vi "average safe rate.vi"(8 "Back Right":dbl, 9 "Front Right":dbl, 10 "Back Left":dbl, 11 "Front Left":dbl) -> (0 "Right Average Rate":dbl, 3 "Left Average Rate":dbl)   [LabVIEW 2014]
panel:
  # "If the person reading this is Michael, haha too late, this was committed\n\nIf the person reading this isn't Michael, hello! From the past!"
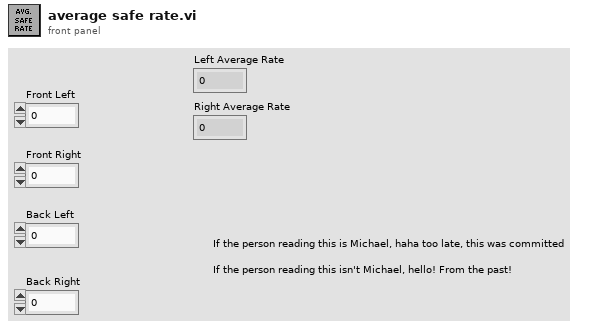
[diagram p1: front panel]
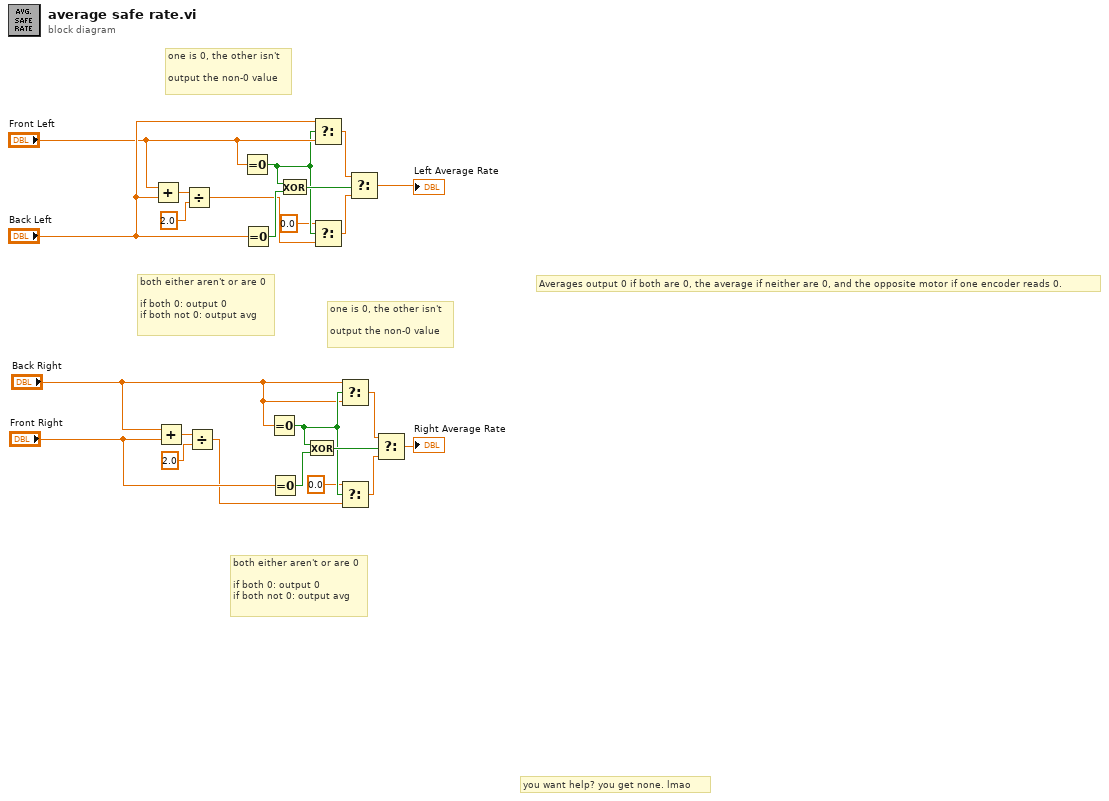
[diagram p0: block diagram]
diagram:
  # "one is 0, the other isn't\n\noutput the non-0 value"
  # "one is 0, the other isn't\n\noutput the non-0 value"
  # "both either aren't or are 0\n\nif both 0: output 0\nif both not 0: output avg"
  # "both either aren't or are 0\n\nif both 0: output 0\nif both not 0: output avg"
  # "Averages output 0 if both are 0, the average if neither are 0, and the opposite motor if one encoder reads 0."
  # "you want help? you get none. lmao"
  n1 = Add(x="Front Left", y="Back Left") -> (x+y=w24:dbl)
  n2 = Add(x="Back Right", y="Front Right") -> (x+y=w21:dbl)
  n3 = Divide(x=w24, y=2.0) -> (x/y=w12:dbl)
  n4 = Divide(x=w21, y=2.0) -> (x/y=w1:dbl)
  n5 = Equal To 0?(x="Front Left") -> (x = 0?=w14:bool)
  n6 = Equal To 0?(x="Back Left") -> (x = 0?=w20:bool)
  n7 = Equal To 0?(x="Back Right") -> (x = 0?=w6:bool)
  n8 = Equal To 0?(x="Front Right") -> (x = 0?=w10:bool)
  n9 = Exclusive Or(1:w20, 2:w14) -> (0:w19:bool)
  n10 = Exclusive Or(1:w10, 2:w6) -> (0:w9:bool)
  n11 = Select(t="Back Left", s=w14, f="Front Left") -> (s? t:f=w16:dbl)
  n12 = Select(t=0.0, s=w14, f=w12) -> (s? t:f=w15:dbl)
  n13 = Select(t="Back Right", s=w6, f="Back Right") -> (s? t:f=w8:dbl)
  n14 = Select(t=0.0, s=w6, f=w1) -> (s? t:f=w7:dbl)
  n15 = Select(t=w16, s=w19, f=w15) -> (s? t:f=→"Left Average Rate":dbl)
  n16 = Select(t=w8, s=w9, f=w7) -> (s? t:f=→"Right Average Rate":dbl)
